vi "Read shift registers.vi"(9 "Loop in":refnum<class "Loop.lvclass">) -> (3 "Loop out":refnum<class "Loop.lvclass">, 4 "shift registers":refnum<class "ShiftRegister.lvclass">[](array[class]))   [LabVIEW 2014, in "Raspberry Pi Compatible Compiler for LabVIEW.lvlib" / "Loop.lvclass"]
uses:
  Loop.lvclass
  ShiftRegister/ShiftRegister.lvclass
  Loop.lvclass/Loop.ctl
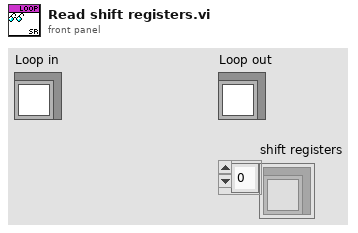
[diagram p1: front panel]
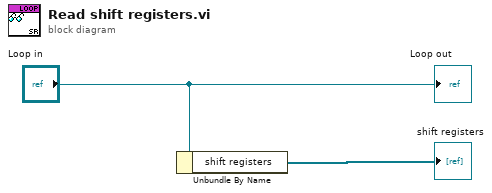
[diagram p0: block diagram]
diagram:
  n1 = Unbundle By Name("Loop in") -> ("shift registers"=→"shift registers":refnum<class "ShiftRegister.lvclass">[])
  "Loop out" <- "Loop in"
